vi "pkt przecięcia prostych.vi"(2 "error in":errorcluster, 3 "Równanie Prostej 2":dbl[](array[numeric]), 4 "Równanie Prostej 1":dbl[](array[numeric])) -> (0 "error out":errorcluster, 1 "Punkt Przecięcia":dbl[](array[numeric]))   [LabVIEW 2016]
doc: "To subvi przyjumuje dwa równania prostych i zwraca punkt ich przecięcia lub bład(error output) jeśli takowy punkt nie istnieje"
uses:
  <vilib>/Analysis/NI_AALBase.lvlib
  <vilib>/Analysis/NI_AALPro.lvlib
  <vilib>/Analysis/baseanly.llb/Matrix Type of Inverse Matrix.ctl
  <vilib>/Analysis/Matrix/NI_Matrix.lvlib
  <vilib>/Analysis/Matrix/Datatypes/RealMatrix.ctl
  <vilib>/Analysis/Matrix/Numeric/Conversions/Matrix To Array - RM.vi
  <vilib>/Analysis/Matrix/Numeric/Conversions/Array To Matrix - RA2.vi
  <vilib>/Analysis/baseanly.llb/Real Determinant.vi
  <vilib>/Analysis/7linalg.llb/Solve Linear Equations (multiple right hand).vi
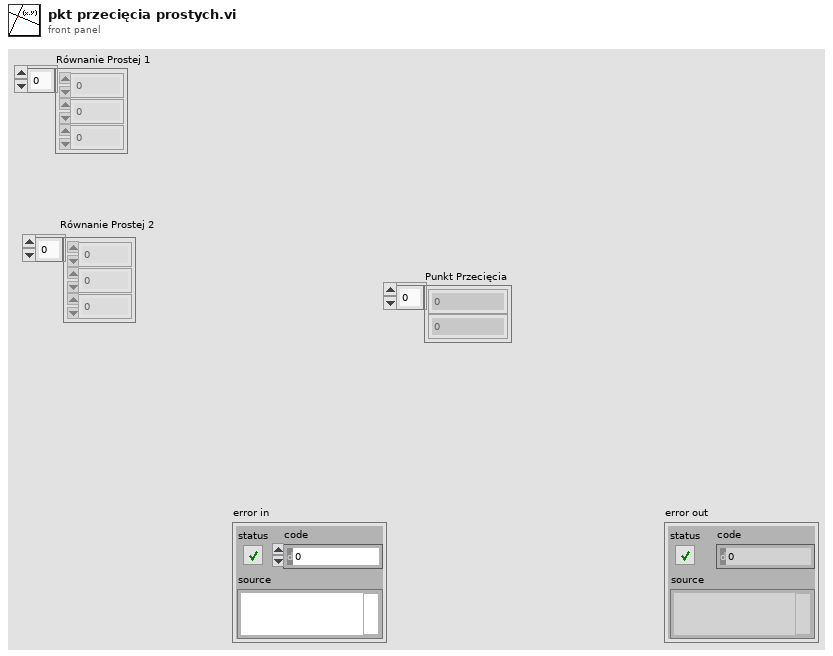
[diagram p1: front panel]
types:
  T1 = typedef "NI_Matrix.lvlib/RealMatrix.ctl" = dbl[][]
  T2 = enum32{"General", "Positive Definite", "Lower Triangular", "Upper Triangular"}
  T3 = typedef "NI_AALBase.lvlib/Matrix Type of Inverse Matrix.ctl" = enum32{"General", "Positive Definite", "Lower Triangular", "Upper Triangular"}
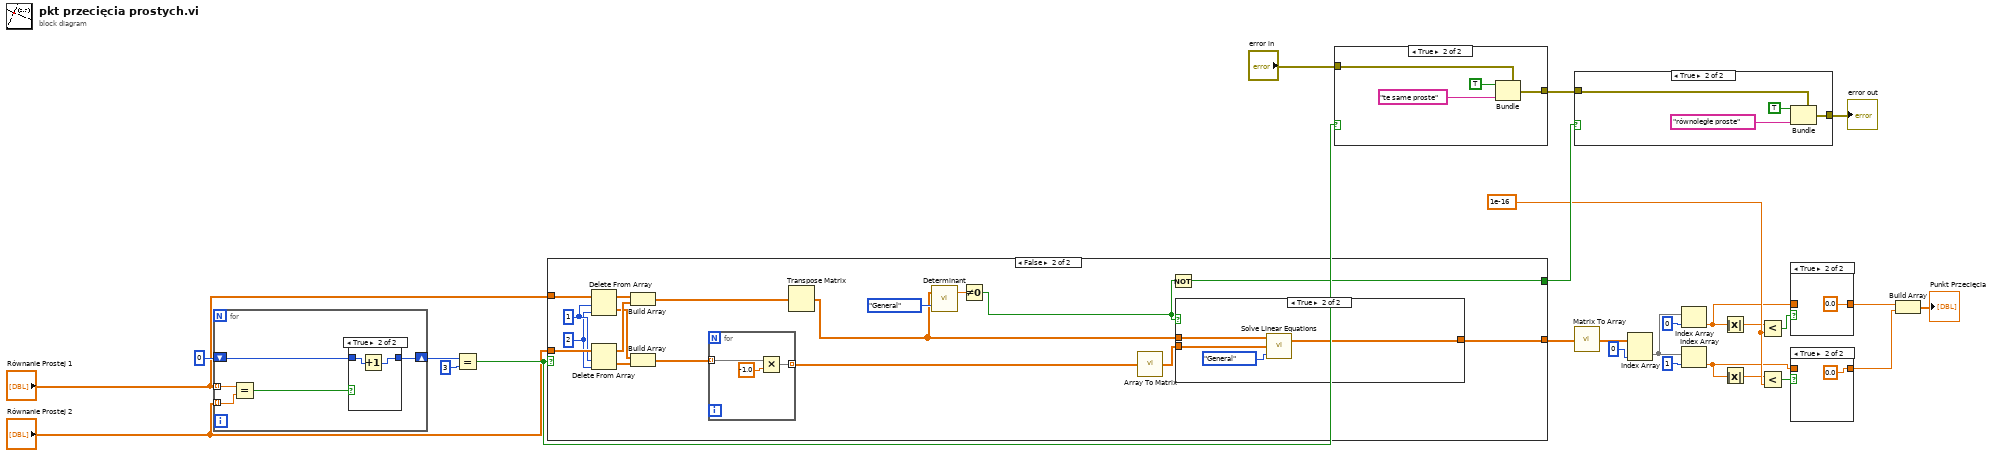
[diagram p0: block diagram]
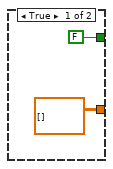
[diagram p4: hidden frame]
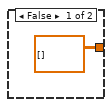
[diagram p5: hidden frame]
diagram:
  w9 = 1e-16
  n1 = for {
    tunnel: "Równanie Prostej 1" -> [w31] mode=indexing
    tunnel: "Równanie Prostej 2" -> [w30] mode=indexing
    shift-right: [w27] -> w20
    shift-left: 0 -> [w28]
    n2 = Equal?(x=w31, y=w30) -> (x = y?=w29:bool)
    n3 = case shown="True" w29 {
      tunnel: w28 -> [w32 w34]
      tunnel: [w32 w33] -> w27
      frame False {
      }
      frame True {
        n4 = Increment(x=w34) -> (x+1=w33:i32)
      }
    }
  }
  n5 = Equal?(x=w20, y=3) -> (x = y?=w19:bool)
  n6 = case shown="False" w19 {
    tunnel: [FALSE w49] -> w25
    tunnel: "Równanie Prostej 1" -> [_ w47]
    tunnel: "Równanie Prostej 2" -> [_ w48]
    tunnel: [T1 [] ("Solution Matrix") w37] -> w18
    frame True {
    }
    frame False {
      w42 = 2 ("index")
      w43 = 1 ("length")
      n7 = Delete From Array(array=w47, length=w43, index=w42) -> (deleted portion=w46:dbl[], array with subset deleted=w54:dbl[])
      n8 = Delete From Array(array=w48, length=w43, index=w42) -> (deleted portion=w45:dbl[], array with subset deleted=w53:dbl[])
      n9 = Build Array(w54, w53) -> (w39:T1)
      n10 = Build Array(w46, w45) -> (w44:dbl[][])
      n11 = for {
        tunnel: w44 -> [w56] mode=indexing
        tunnel: [w55] -> w41 mode=indexing
        n12 = Multiply(x=w56, y=-1.0) -> (x*y=w55:dbl[])
      }
      n13 = Transpose Matrix(1:w39) -> (0:w38:T1)
      n14 = call-poly <vilib>:"Determinant.vi"("matrix type"=T2."General", "Input Matrix"=w38) -> ("determinant"=w52:dbl)  [unwired: 1 out]
      n15 = Not Equal To 0?(x=w52) -> (x != 0?=w50:bool)
      n16 = call-poly <vilib>:"Array To Matrix.vi"("Real 2D Array"=w41) -> ("Real Matrix"=w40:T1)
      n17 = Not(x=w50) -> (.not. x?=w49:bool)
      n18 = case shown="True" w50 {
        tunnel: w38 -> [_ w62]
        tunnel: w40 -> [_ w61]
        tunnel: [T1 [] ("Solution Matrix") w59] -> w37
        frame False {
        }
        frame True {
          n19 = call-poly <vilib>:"Solve Linear Equations.vi"("matrix type"=Matrix_Type_of_Inverse_Matrix."General", "Known Matrix"=w61, "Input Matrix"=w62) -> ("Solution Matrix"=w59:T1)  [unwired: 1 out]
        }
      }
    }
  }
  n20 = case shown="True" w19 {
    tunnel: [w63 w64] -> w24
    tunnel: "error in" -> [w63 w65]
    frame False {
    }
    frame True {
      n21 = Bundle(cluster=w65, "status"=TRUE, "source"="te same proste") -> (w64:errorcluster)  [unwired: 1 in]
    }
  }
  n22 = case shown="True" w25 {
    tunnel: w24 -> [w68 w70]
    tunnel: [w68 w69] -> w26
    frame False {
    }
    frame True {
      n23 = Bundle(cluster=w70, "status"=TRUE, "source"="równoległe proste") -> (w69:errorcluster)  [unwired: 1 in]
    }
  }
  "error out" <- w26
  n24 = call-poly <vilib>:"Matrix To Array.vi"("Real Matrix"=w18) -> ("Real 2D Array"=w17:dbl[][])
  n25 = Index Array(array=w17, index (col)=0 ("disabled index (col)")) -> (element=w13:dbl[])  [unwired: 1 in]
  n26 = Index Array(array=w13, index=0) -> (element=w4:dbl)
  n27 = Index Array(array=w13, index=1) -> (element=w2:dbl)
  n28 = Absolute Value(x=w4) -> (abs(x)=w3:dbl)
  n29 = Absolute Value(x=w2) -> (abs(x)=w1:dbl)
  n30 = Less?(x=w3, y=w9) -> (x < y?=w10:bool)
  n31 = Less?(x=w1, y=w9) -> (x < y?=w8:bool)
  n32 = case shown="True" w10 {
    tunnel: [w73 0.0 ("element")] -> w7
    tunnel: w4 -> [w73 _]
    frame False {
    }
    frame True {
    }
  }
  n33 = case shown="True" w8 {
    tunnel: [w75 0.0] -> w6
    tunnel: w2 -> [w75 _]
    frame False {
    }
    frame True {
    }
  }
  n34 = Build Array(w7, w6) -> (→"Punkt Przecięcia":dbl[])
